vi "Finish.vi"   [LabVIEW 2017]
doc: "This VI is called just before exiting. It is expected to close I/O refnum, save collected data, etc."
uses:
  Globals/Global_STOP.vi
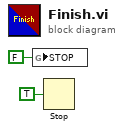
[diagram p0: block diagram]
diagram:
  n1 = global write "Global_STOP.vi" "STOP"(FALSE ("STOP")) -> ()
  n2 = Stop(stop? (T)=TRUE) -> ()
